vi "stopwatchSpinner.vi"(9 "notifier":refnum<notifier>, 11 "displayText":string) -> ()   [LabVIEW 2022 SP3]
panel:
  out "message":string
  out "elapsedTime":cluster{"Numeric":dbl, "Numeric":dbl}(knob)={"Numeric"=0.0, "Numeric"=1.1524910234112342} scale=0.0..100.0
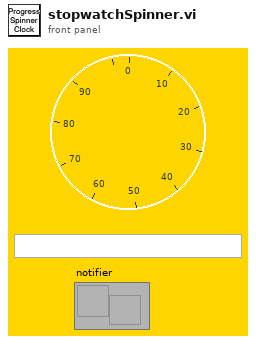
[diagram p1: front panel]
types:
  T1 = enum32{"Invalid", "Standard", "Closed", "Hidden", "Minimized", "Maximized"}
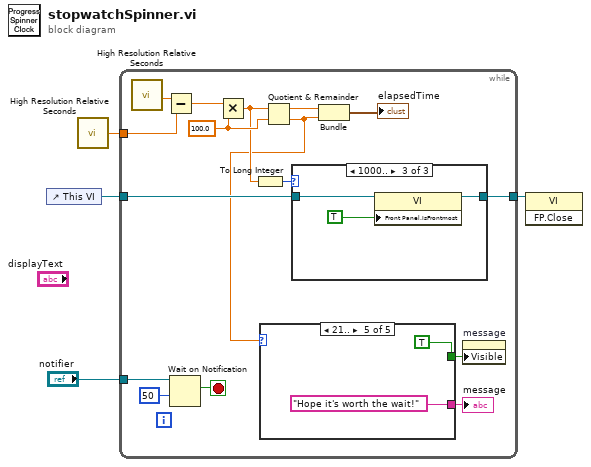
[diagram p0: block diagram]
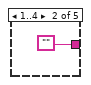
[diagram p3: hidden frame]
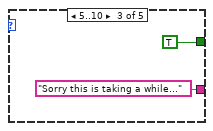
[diagram p4: hidden frame]
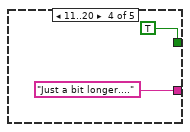
[diagram p5: hidden frame]
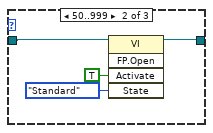
[diagram p7: hidden frame]
diagram:
  n1 = control-ref of="This VI"() -> (w1:refnum<vi>)
  n2 = call <vilib>:"High Resolution Relative Seconds.vi"() -> ("relative seconds"=w3:dbl)
  n3 = while {
    tunnel: "notifier" -> [w18]
    tunnel: w3 -> [w13]
    tunnel: w1 -> [w10]
    tunnel: [w15] -> w2
    stop <- w16 stop-if-true
    w11 = 100.0 ("y")
    n4 = call <vilib>:"High Resolution Relative Seconds.vi"() -> ("relative seconds"=w14:dbl)
    n5 = Subtract(x=w14, y=w13) -> (x-y=w12:dbl)
    n6 = Wait on Notification(notifier=w18, timeout in ms (-1)=u32 50 ("milliseconds to wait")) -> (notification=w16:bool)  [unwired: 2 in, 3 out]
    n7 = Multiply(x=w12, y=w11) -> (x*y=w9:dbl)
    n8 = To Long Integer(number=w9) -> (32bit integer=w5:i32)
    n9 = Quotient & Remainder(x=w9, y=w11) -> (x-y*floor(x/y)=w20:dbl, floor(x/y)=w7:dbl)
    n10 = case shown="21.." w7 {
      tunnel: [_ "" "Sorry this is taking a while..." "Just a bit longer...." "Hope it's worth the wait!"] -> w8
      tunnel: [_ _ TRUE ("Visible") TRUE ("Visible") TRUE ("Visible")] -> w6
      frame 0, Default {
      }
      frame 1..4 {
      }
      frame 5..10 {
      }
      frame 11..20 {
      }
      frame 21.. {
      }
    }
    "message" <- w8
    n11 = case shown="1000.." w5 {
      tunnel: [w28 w29 w34] -> w15
      tunnel: w10 -> [w28 w30 w35]
      frame 0, Default {
      }
      frame 50..999 {
        n12 = invoke class="VI" method="FP.Open"(reference=w30, "Activate"=TRUE ("Activate?"), "State"=T1."Standard") -> (reference out=w29:refnum<vi>)  [unwired: 2 in, 4 out]
      }
      frame 1000.. {
        n13 = property class="VI"(reference=w35, "Front Panel.IsFrontmost"=TRUE ("Activate?")) -> (reference out=w34:refnum<vi>)  [unwired: 1 in, 1 out]
      }
    }
    n14 = Bundle(w20, w7) -> (→"elapsedTime":cluster{dbl, dbl})  [unwired: 1 in]
    n15 = property on="message" class="Str"("Visible"=w6) -> ()  [unwired: 2 in, 2 out]
  }
  n16 = invoke class="VI" method="FP.Close"(reference=w2) -> ()  [unwired: 2 in, 3 out]
